vi "Reset Wheels.vi"() -> ()   [LabVIEW 2016]
uses:
  Refname/Motors.ctl
  Refname/Refname to String (Motors).vi
  <vilib>/addons/control/pid/pid.llb/PID (DBL).vi
  <vilib>/addons/control/pid/NI_PID_pid.lvlib
panel:
  in  "output range":cluster{"output high":dbl, "output low":dbl}={"output high"=100.0, "output low"=-100.0} {"output low" format="%.2f"; "output high" format="%.2f"}
  in  "Tolerance":dbl format="%#_13g"
  in  "PID gains":T1={"proportional gain (Kc)"=1.0, "integral time (Ti, min)"=0.01, "derivative time (Td, min)"=0.0} {"derivative time (Td, min)" format="%.3f"; "integral time (Ti, min)" format="%.8f"; "proportional gain (Kc)" format="%.8f"}
  in  "Setpoint":i32
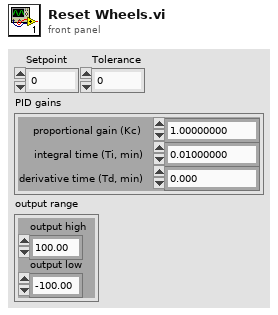
[diagram p1: front panel]
types:
  T1 = cluster{"proportional gain (Kc)":dbl, "integral time (Ti, min)":dbl, "derivative time (Td, min)":dbl}
  T2 = typedef "Motors.ctl" = enum16{"Wheel 1", "Swerve 1", "Wheel 2", "Swerve 2", "Wheel 3", "Swerve 3", "Wheel 4", "Swerve 4"}
  T3 = typedef "WPI_MotorControlDeviceRef.ctl" = cluster{"DeviceStatus":errorcluster, "Type":T4, "PWM":cluster{"PWM Channel":T5, "DeadBand":T6}, "CAN":cluster{"Device Number":u8, "SetOutput VI Ref":variant, "GetOutput VI Ref":variant, "Enable VI Ref":variant, "Disable VI Ref":variant, "Data":variant}, "Invert":bool}
  T4 = typedef "WPI_MotorControlType.ctl" = enum16{"PWM", "CAN"}
  T5 = typedef "FPGA_DIOPWMChannel.ctl" = enum8{"PWM 0", "PWM 1", "PWM 2", "PWM 3", "PWM 4", "PWM 5", "PWM 6", "PWM 7", "PWM 8", "PWM 9", "PWM MXP 0", "PWM MXP 1", "PWM MXP 2", "PWM MXP 3", "PWM MXP 4", "PWM MXP 5", "PWM MXP 6", "PWM MXP 7", "PWM MXP 8", "PWM MXP 9", "Invalid"}
  T6 = typedef "WPI_PWMDeadband.ctl" = cluster{"Name":string, "maxPositivePwm":i32, "minPositivePwm":i32, "centerPwm":i32, "maxNegativePwm":i32, "minNegativePwm":i32, "angularRange":u16}
  T7 = typedef "WPI_CANTalonSRX_GlobalStatus.ctl" = cluster{"Applied Throttle":dbl, "Module Enabled":bool, "CAN Error":errorcluster, "Closed Loop Error":dbl, "Forward Limit Switch Closed":bool, "Reverse Limit Switch Closed":bool, "Sensor Position":dbl, "Sensor Velocity":dbl, "Current":dbl, "Sticky Fault - Over Temp":bool, "Sticky Fault - Under Voltage":bool, "Sticky Fault - Forward Limit":bool, "Sticky Fault - Reverse Limit":bool, "Sticky Fault - Forward Soft Limit":bool, "Sticky Fault - Reverse Soft Limit":bool, "Brake is Enabled":bool, "Encoder Position":dbl, "Encoder Velocity":dbl, "Encoder Index Count":dbl, "Encoder A Pin State":bool, "Encoder B Pin State":bool, "Encoder Index Pin State":bool, "Analog In":dbl, "Analog In Velocity":dbl, "Temperature (C)":dbl, "Battery Voltage":dbl, "Control 5 Is Supported":bool, "Current Profile Slot Select":dbl, "Pos Div 8":bool, "Vel Div 4":bool, "Pulse Width Position":i32, "Pulse Width Velocity":i32, "Pulse Width Rise To Rise (us)":i32, "Pulse Width Rise To Fall (us)":i32, "Mot Prof Active Is Under Run":bool, "Mot Prof Active Has Under Run":bool, "Mot Prof Active Is Last":bool, "Mot Prof Active Velocity Only":bool, "Mot Prof Active Is Valid":bool, "Mot Prof Buffer Is Full":bool, "Mot Prof Active Profile Slot Select":i32, "Mot Prof NextID":i32, "Mot Prof Count":i32, "Mot Prof Active Velocity":dbl, "Mot Prof Active Position":dbl, "Mot Prof Output Enable":i32}
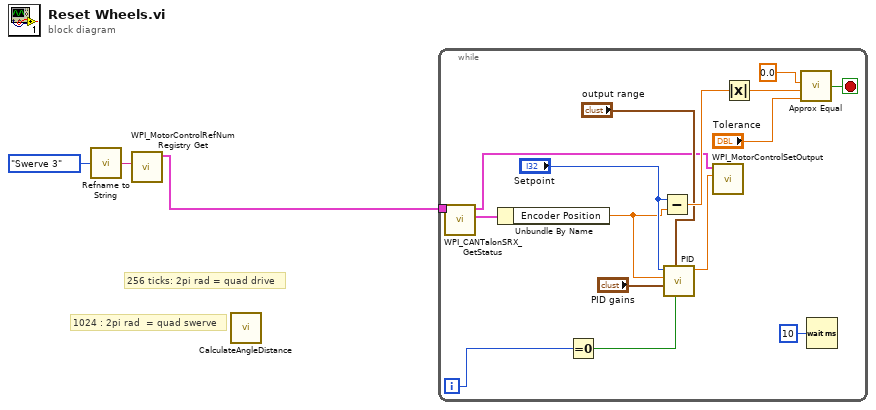
[diagram p0: block diagram]
diagram:
  # "1024 : 2pi rad  = quad swerve"
  # "256 ticks: 2pi rad = quad drive"
  n1 = call-poly "Refname to String.vi"("Enum"=Motors."Swerve 3") -> ("String"=w2:string)
  n2 = call <vilib>:"WPI_MotorControlRefNum Registry Get.vi"("refnum name"=w2) -> ("MotorControlDevRef"=w1:T3)  [unwired: 9 in, 1 out]
  n3 = call "CalculateAngleDistance.vi"() -> ()  [unwired: 11 in, 1 out]
  n4 = while {
    tunnel: w1 -> [w9]
    i -> [w5]
    stop <- w17 stop-if-true
    n5 = call <vilib>:"WPI_CANTalonSRX_GetStatus.vi"("CAN Talon SRX Ref"=w9) -> ("Talon SRX Status"=w10:T7, "CAN Talon SRX Ref"=w7:T3)  [unwired: 8 in, 1 out]
    n6 = Unbundle By Name(w10) -> ("Encoder Position"=w8:dbl)
    n7 = Equal To 0?(x=w5) -> (x = 0?=w4:bool)
    n8 = Subtract(x="Setpoint", y=w8) -> (x-y=w15:dbl)
    n9 = call-poly <vilib>:"PID.vi"("reinitialize? (F)"=w4, "output range"="output range", "PID gains"="PID gains", "process variable"=w8, "setpoint"="Setpoint") -> ("output"=w18:dbl)  [unwired: 5 in, 1 out]
    n10 = call <vilib>:"WPI_MotorControlSetOutput.vi"("Output"=w18, "MotorControlDevRef"=w7) -> ()  [unwired: 7 in, 3 out]
    n11 = Absolute Value(x=w15) -> (abs(x)=w14:dbl)
    n12 = call "Approx Equal.vi"("Tolerance"="Tolerance", "b"=w14, "a"=0.0) -> ("a == b?"=w17:bool)  [unwired: 1 in]
    n13 = Wait (ms)(milliseconds to wait=u32 10) -> ()  [unwired: 1 out]
  }
